vi "Tarea 6.vi"() -> ()   [LabVIEW 2019]
uses:
  Student Material/Student Material/Module 2/Exercise 6/CLD 6 CSV file data structure.ctl
  <vilib>/Utility/file.llb/Read Delimited Spreadsheet (string).vi
  Student Material/Student Material/Module 2/Exercise 6/CLD 6 CSV file enum.ctl
panel:
  out "Error Out":errorcluster
  in  "Error In":errorcluster
  in  "[Data In]":T1[](array[typedef])=[{"Dwell Time"=3, "State 1"=TRUE, "State 2"=FALSE, "State 3"=FALSE}, {"Dwell Time"=4, "State 1"=FALSE, "State 2"=TRUE, "State 3"=FALSE}, {"Dwell Time"=5, "State 1"=FALSE, "State 2"=FALSE, "State 3"=TRUE}]
  in  "Read/ Write":T2
  out "[Data Out]":T1[](array[typedef])
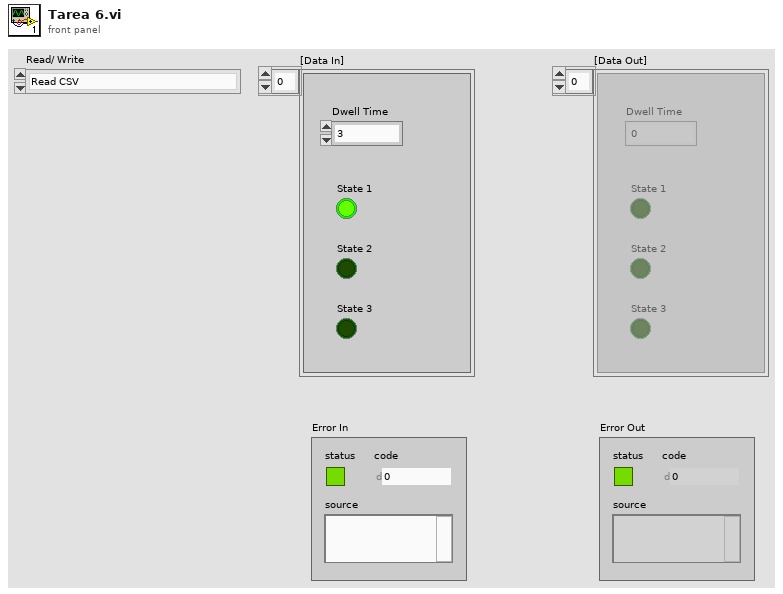
[diagram p1: front panel]
types:
  T1 = typedef "CLD 6 CSV file data structure.ctl" = cluster{"Dwell Time":i32, "State 1":bool, "State 2":bool, "State 3":bool}
  T2 = typedef "CLD 6 CSV file enum.ctl" = enum16{"Read CSV", "Write CSV"}
  T3 = enum16{"open", "replace", "create", "open or create", "replace or create", "replace or create with confirmation"}
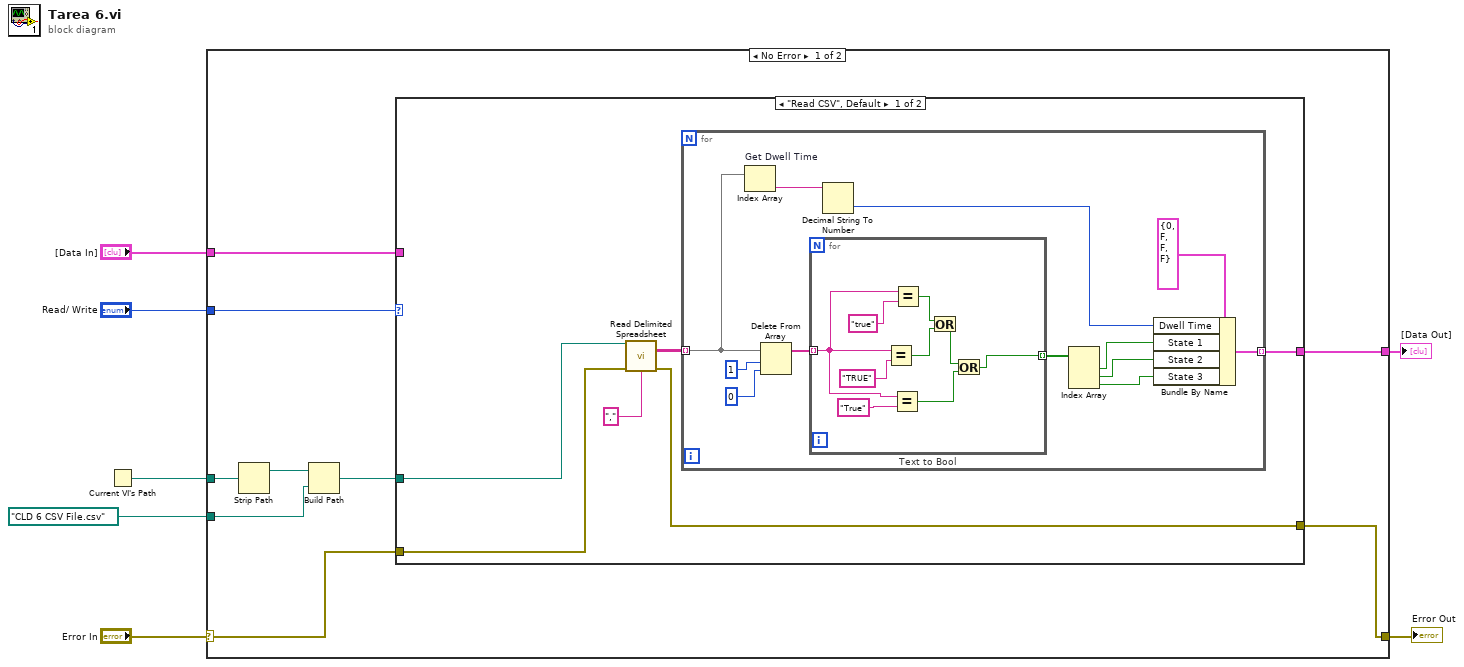
[diagram p0: block diagram]
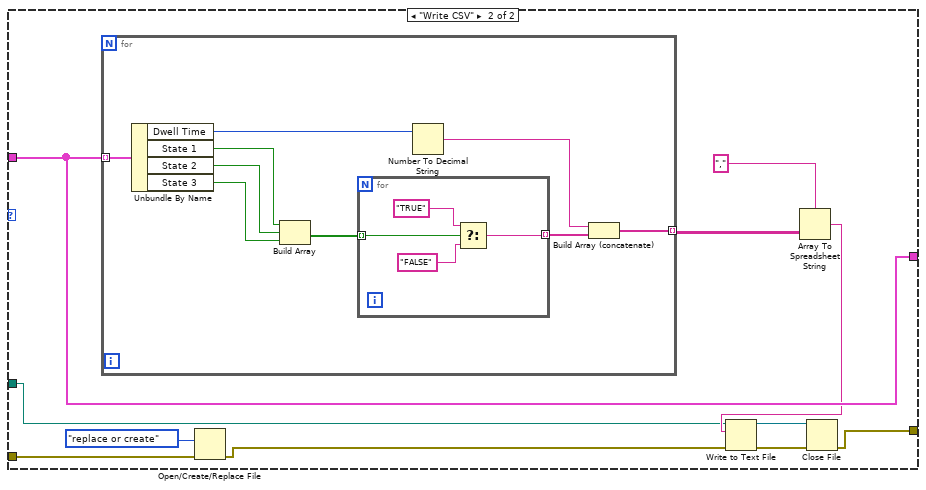
[diagram p2: hidden frame]
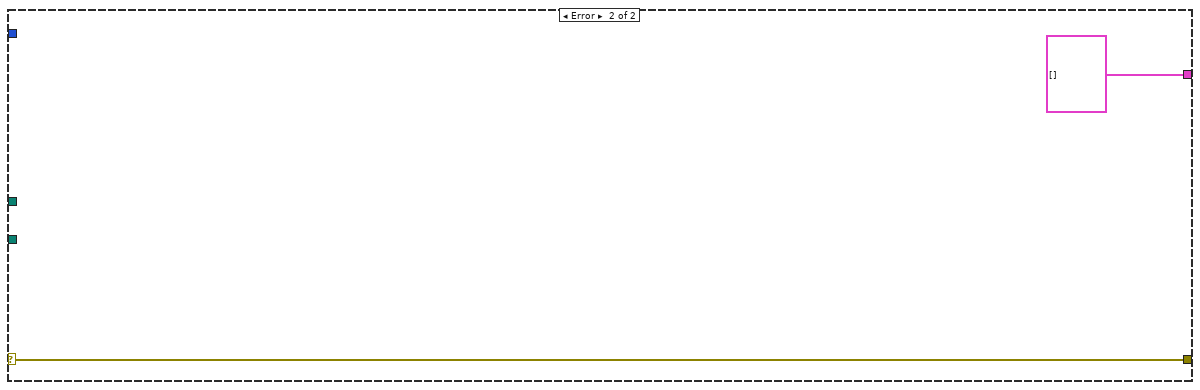
[diagram p3: hidden frame]
diagram:
  n1 = Current VI's Path() -> (path=w5:path)
  n2 = case shown="No Error" "Error In" {
    selector: "Error In" -> [w9 w69]
    tunnel: [w16 T1[] [] ("[Data In]")] -> w7
    tunnel: path "CLD 6 CSV File.csv" -> [w15 _]
    tunnel: w5 -> [w14 _]
    tunnel: "Read/ Write" -> [w12 _]
    tunnel: "[Data In]" -> [w11 _]
    tunnel: [w8 w69] -> w1
    frame No Error {
      n3 = Strip Path(path=w14) -> (stripped path=w10:path)  [unwired: 1 out]
      n4 = Build Path(base path=w10, name or relative path=w15) -> (appended path=w13:path)
      n5 = case shown="\"Read CSV\", Default" w12 {
        tunnel: w13 -> [w22 w44]
        tunnel: [w21 w54] -> w16
        tunnel: w11 -> [_ w54]
        tunnel: w9 -> [w18 w51]
        tunnel: [w17 w47] -> w8
        frame "Read CSV", Default {
          n6 = call-poly <vilib>:"Read Delimited Spreadsheet.vi"("file path (dialog if empty)"=w22, "error in (no error)"=w18, "delimiter (\\t)"="," ("delimiter (\\t)")) -> ("all rows"=w19:string[][], "error out"=w17:errorcluster)  [unwired: 7 in, 4 out]
          n7 = for {
            tunnel: w19 -> [w31] mode=indexing
            tunnel: [w34] -> w21 mode=indexing
            n8 = Index Array "Get Dwell Time"(array=w31) -> (element=w33:string)  [unwired: 1 in]
            n9 = Delete From Array(array=w31, length=1, index=0) -> (array with subset deleted=w24:string[])  [unwired: 1 out]
            n10 = for "Text to Bool" {
              tunnel: w24 -> [w36] mode=indexing
              tunnel: [w39] -> w28 mode=indexing
              n11 = Equal?(x=w36, y="TRUE") -> (x = y?=w42:bool)
              n12 = Equal?(x=w36, y="True") -> (x = y?=w40:bool)
              n13 = Equal?(x=w36, y="true") -> (x = y?=w35:bool)
              n14 = Or(x=w35, y=w42) -> (x .or. y?=w41:bool)
              n15 = Or(x=w41, y=w40) -> (x .or. y?=w39:bool)
            }
            n16 = Decimal String To Number(string=w33) -> (number=w32:i32)  [unwired: 2 in, 1 out]
            n17 = Index Array(array=w28) -> (element #1=w27:bool, element #2=w26:bool, element #3=w25:bool)  [unwired: 3 in]
            n18 = Bundle By Name(cluster=T1 {"Dwell Time"=0, "State 1"=FALSE, "State 2"=FALSE, "State 3"=FALSE} ("CSV File Data Structure"), "Dwell Time"=w32, "State 1"=w27, "State 2"=w26, "State 3"=w25) -> (w34:T1)
          }
        }
        frame "Write CSV" {
          n19 = for {
            tunnel: w54 -> [w63] mode=indexing
            tunnel: [w55] -> w52 mode=indexing
            n20 = Unbundle By Name(w63) -> ("Dwell Time"=w62:i32, "State 1"=w61:bool, "State 2"=w60:bool, "State 3"=w59:bool)
            n21 = Build Array(w61, w60, w59) -> (w58:bool[])
            n22 = for {
              tunnel: w58 -> [w67] mode=indexing
              tunnel: [w64] -> w56 mode=indexing
              n23 = Select(t="TRUE", s=w67, f="FALSE") -> (s? t:f=w64:string)
            }
            n24 = Number To Decimal String(number=w62) -> (decimal integer string=w57:string)  [unwired: 1 in]
            n25 = Build Array (concatenate)(w57, w56) -> (w55:string[])
          }
          n26 = Open/Create/Replace File(error in=w51, operation (0:open)=T3."replace or create") -> (error out=w46:errorcluster)  [unwired: 4 in, 2 out]
          n27 = Array To Spreadsheet String(delimiter (Tab)="," ("delimiter (\\t)"), array=w52) -> (spreadsheet string=w45:string)  [unwired: 1 in]
          n28 = Write to Text File(file (use dialog)=w44, text=w45, error in=w46) -> (refnum out=w48:refnum<file>, error out=w49:errorcluster)  [unwired: 1 in, 1 out]
          n29 = Close File(refnum=w48, error in=w49) -> (error out=w47:errorcluster)  [unwired: 1 out]
        }
      }
    }
    frame Error {
    }
  }
  "[Data Out]" <- w7
  "Error Out" <- w1
